vi "JAC_8216_Setting_Function_New.vi"(0 "JAC 8216_Control":T5, 1 "Initial":T4={"Card ID"=0, "IP_Address[4]"=[192, 168, 0, 100], "Hot post"=15122, "Remote port"=6936, "Time Out(ms)"=1000} {"Card ID" items=["0", "1", "2", "3", "4", "5", "6", "7", "8", "9", "10", "11", "12", "13", "14", "15", "16", "17", "18", "19", "20", "21", "22", "23", "24", "25", "26", "27", "28", "29", "30", "31", "32", "33", "34", "35", "36", "37", "38", "39", "40", "41", "42", "43", "44", "45", "46", "47", "48", "49", "50", "51", "52", "53", "54", "55", "56", "57", "58", "59", "60", "61", "62", "63", "64", "65", "66", "67", "68", "69", "70", "71", "72", "73", "74", "75", "76", "77", "78", "79", "80", "81", "82", "83", "84", "85", "86", "87", "88", "89", "90", "91", "92", "93", "94", "95", "96", "97", "98", "99", "100"]}, 2 "8216 IO In":T3, 3 "IO Polarity In":T1, 4 "IO Config In":T2 {"IO 17" items=["Output", "Input"]; "IO 16" items=["Output", "Input"]; "IO 15" items=["Output", "Input"]; "IO 14" items=["Output", "Input"]; "IO 13" items=["Output", "Input"]; "IO 12" items=["Output", "Input"]; "IO 11" items=["Output", "Input"]; "IO 10" items=["Output", "Input"]; "IO 07" items=["Output", "Input"]; "IO 06" items=["Output", "Input"]; "IO 05" items=["Output", "Input"]; "IO 04" items=["Output", "Input"]; "IO 03" items=["Output", "Input"]; "IO 02" items=["Output", "Input"]; "IO 01" items=["Output", "Input"]; "IO 00" items=["Output", "Input"]}, 5 "Error in":errorcluster) -> (15 "Port Status Out":bool[](array[boolean]), 16 "Input Out":u8, 17 "IO Polarity Out":T1, 18 "IO Config Out":T2 {"IO 17" items=["Output", "Input"]; "IO 16" items=["Output", "Input"]; "IO 15" items=["Output", "Input"]; "IO 14" items=["Output", "Input"]; "IO 13" items=["Output", "Input"]; "IO 12" items=["Output", "Input"]; "IO 11" items=["Output", "Input"]; "IO 10" items=["Output", "Input"]; "IO 07" items=["Output", "Input"]; "IO 06" items=["Output", "Input"]; "IO 05" items=["Output", "Input"]; "IO 04" items=["Output", "Input"]; "IO 03" items=["Output", "Input"]; "IO 02" items=["Output", "Input"]; "IO 01" items=["Output", "Input"]; "IO 00" items=["Output", "Input"]}, 19 "Error Out":errorcluster)   [LabVIEW 2015]
uses:
  JAC_8216_Control.ctl
  EMD8216_64/EMD8216_64.lvlib
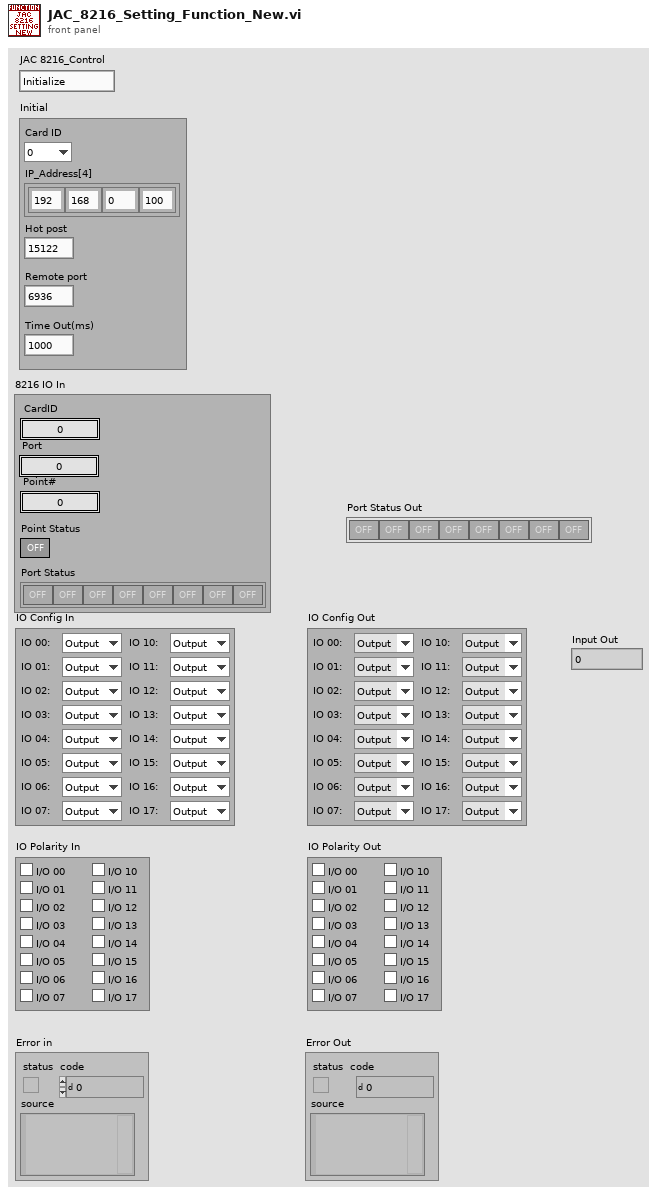
[diagram p1: front panel]
types:
  T1 = cluster{"IO 00":bool, "IO 01":bool, "IO 02":bool, "IO 03":bool, "IO 04":bool, "IO 05":bool, "IO 06":bool, "IO 07":bool, "IO 10":bool, "IO 11":bool, "IO 12":bool, "IO 13":bool, "IO 14":bool, "IO 15":bool, "IO 16":bool, "IO 17":bool}
  T2 = cluster{"IO 00":u8, "IO 01":u8, "IO 02":u8, "IO 03":u8, "IO 04":u8, "IO 05":u8, "IO 06":u8, "IO 07":u8, "IO 10":u8, "IO 11":u8, "IO 12":u8, "IO 13":u8, "IO 14":u8, "IO 15":u8, "IO 16":u8, "IO 17":u8}
  T3 = cluster{"CardID":u32, "Port":u8, "Point#":u8, "Point Status":bool, "Port Status":bool[]}
  T4 = cluster{"Card ID":u32, "IP_Address[4]":u8[], "Hot post":u16, "Remote port":u16, "Time Out(ms)":u16}
  T5 = typedef "JAC_8216_Control.ctl" = enum16{"Initialize", "Log Password", "Read IO Polarity ", "Set IO Polarity", "Read IO Config", "Set IO Config", "Read Input", "Set Output", "Read Port", "Close", "Idle"}
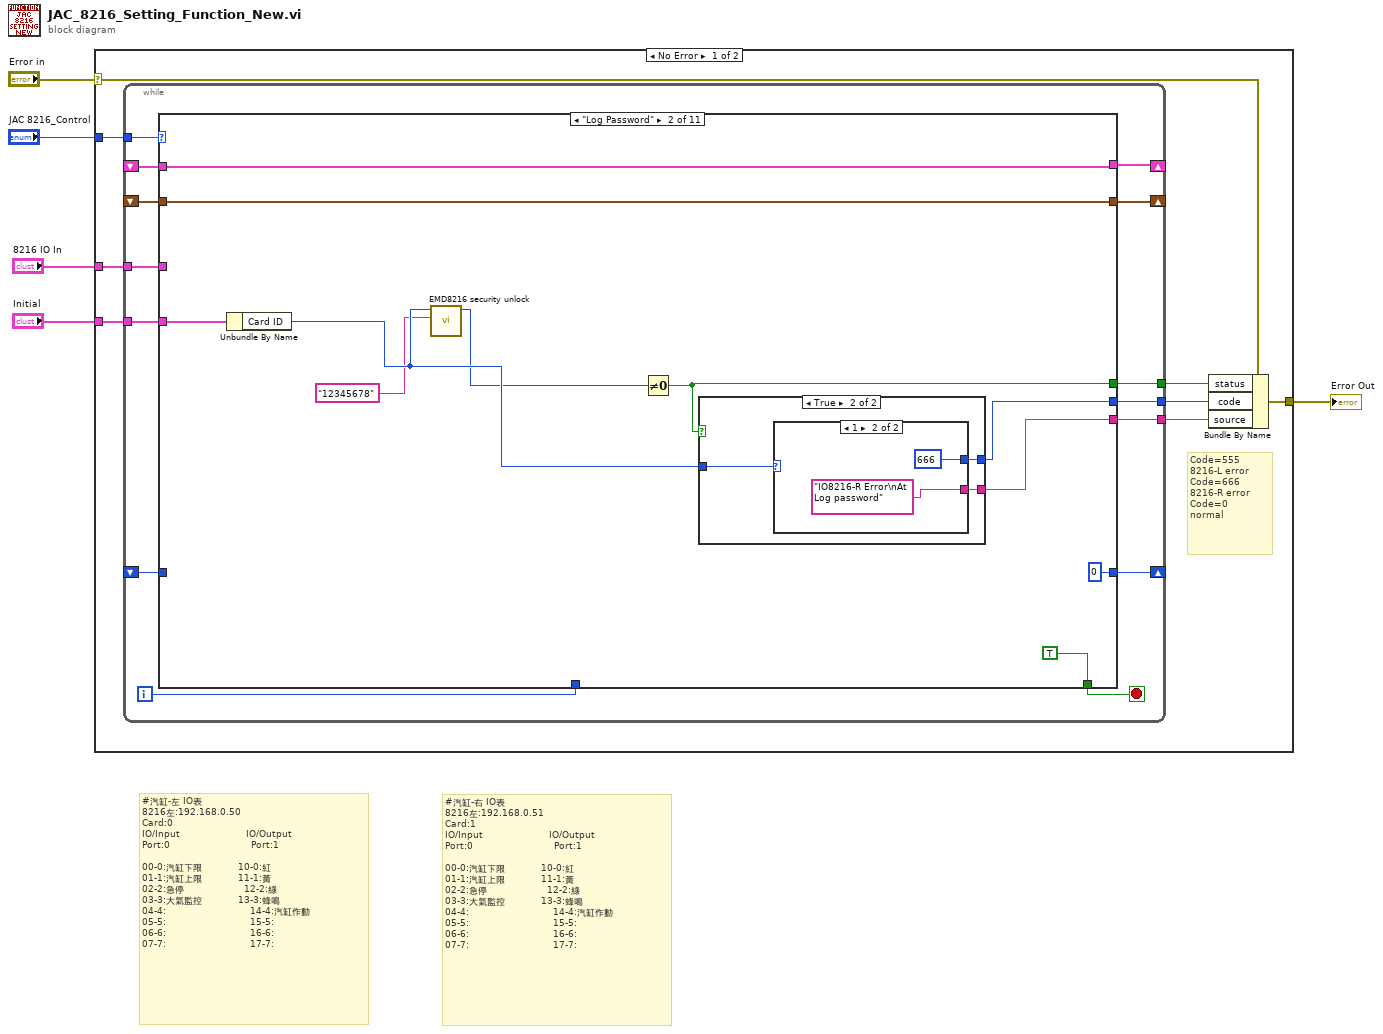
[diagram p0: block diagram]
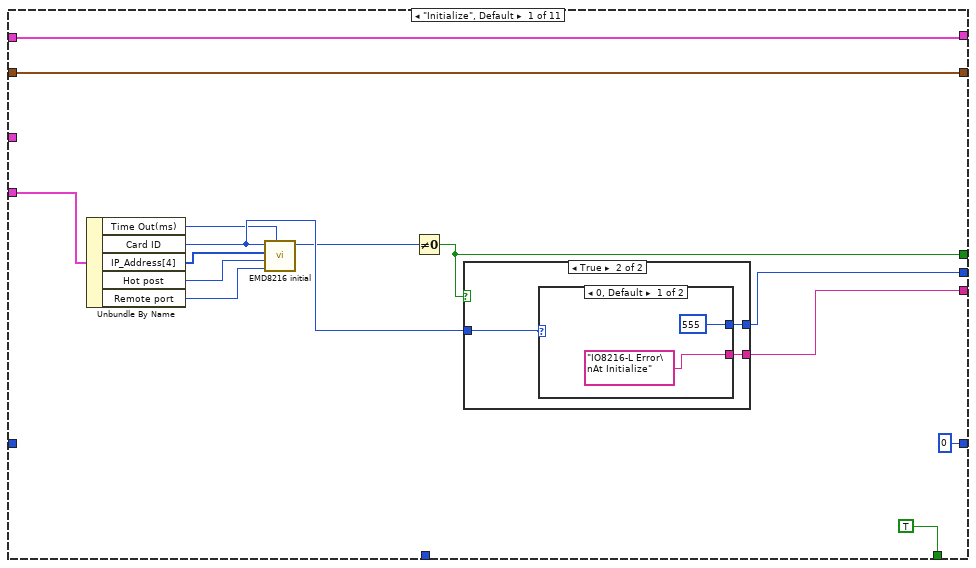
[diagram p2: hidden frame]
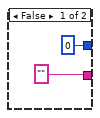
[diagram p3: hidden frame]
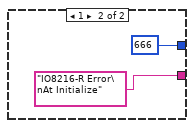
[diagram p4: hidden frame]
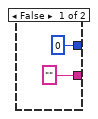
[diagram p5: hidden frame]
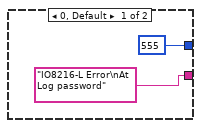
[diagram p6: hidden frame]
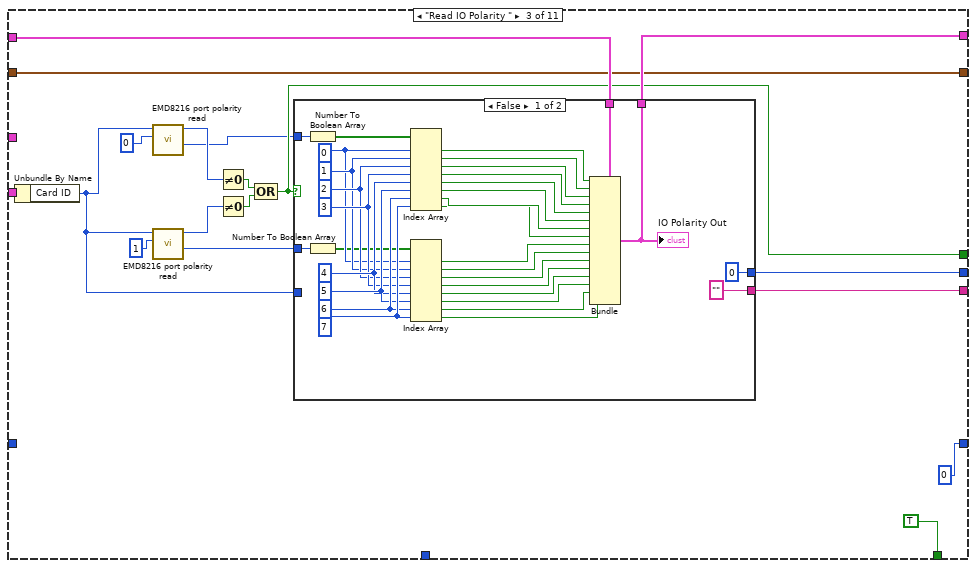
[diagram p7: hidden frame]
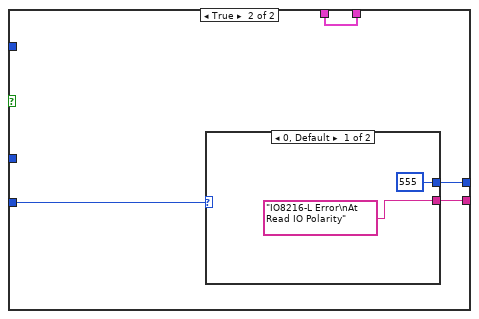
[diagram p8: hidden frame]
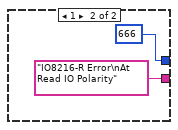
[diagram p9: hidden frame]
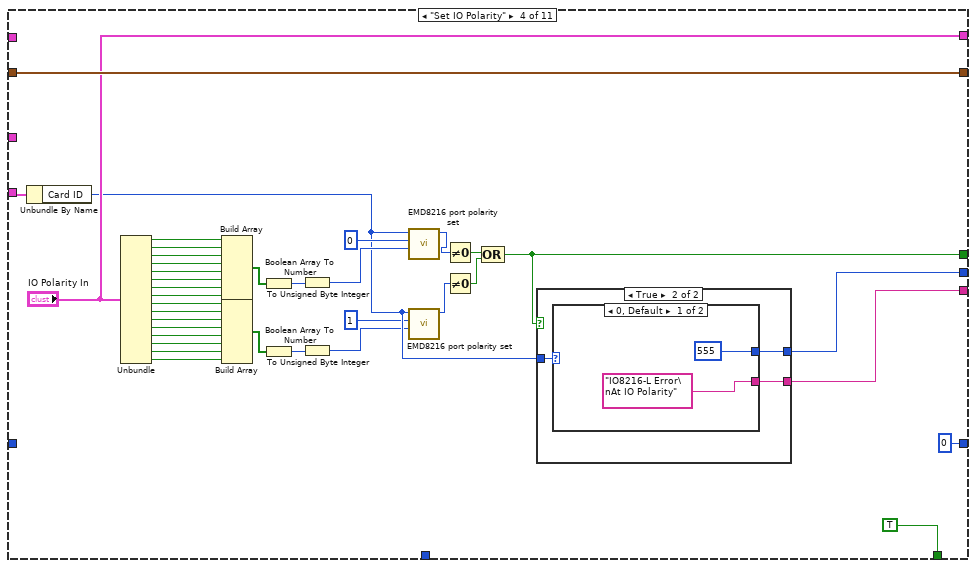
[diagram p10: hidden frame]
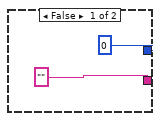
[diagram p11: hidden frame]
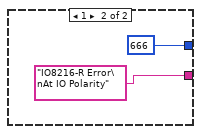
[diagram p12: hidden frame]
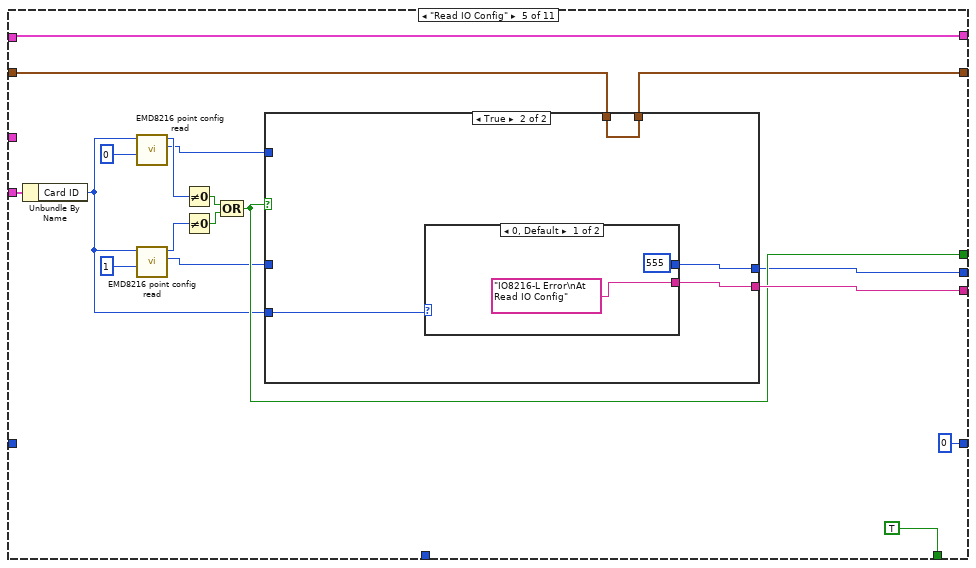
[diagram p13: hidden frame]
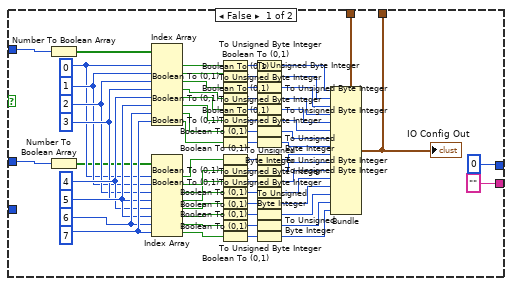
[diagram p14: hidden frame]
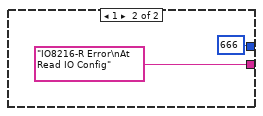
[diagram p15: hidden frame]
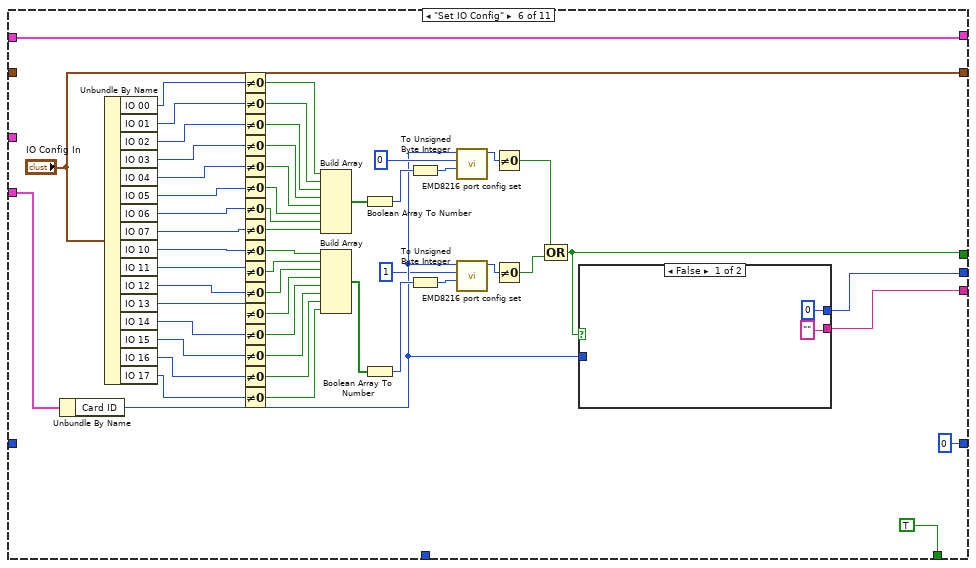
[diagram p16: hidden frame]
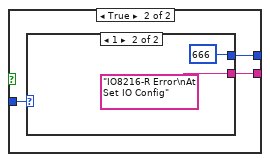
[diagram p17: hidden frame]
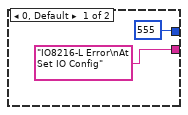
[diagram p18: hidden frame]
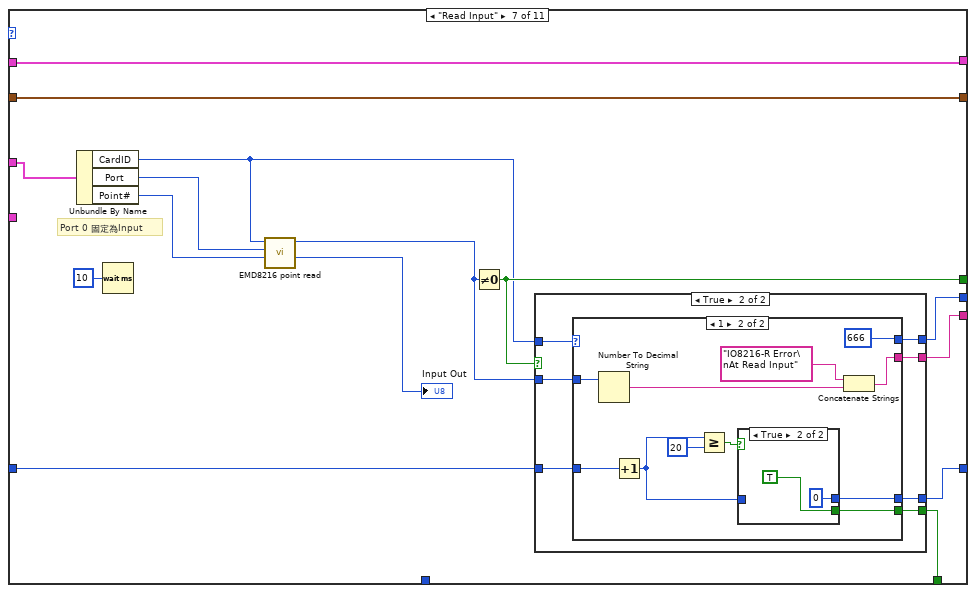
[diagram p19: hidden frame]
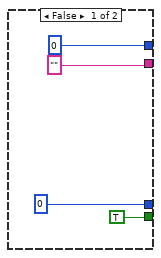
[diagram p20: hidden frame]
diagram:
  # "#汽缸-右 IO表\n8216左:192.168.0.51\nCard:1\nIO/Input                      IO/Output\nPort:0                           Port:1         \n         \n00-0:汽缸下限            10-0:紅   \n01-1:汽缸上限            11-1:黃\n02-2:急停                    12-2:綠\n03-3:大氣監控            13-3:蜂鳴\n04-4:                            14-4:汽缸作動\n05-5:                            15-5:\n06-6:                            16-6:\n07-7:                            17-7:"
  # "#汽缸-左 IO表\n8216左:192.168.0.50\nCard:0\nIO/Input                      IO/Output\nPort:0                           Port:1         \n         \n00-0:汽缸下限            10-0:紅   \n01-1:汽缸上限            11-1:黃\n02-2:急停                    12-2:綠\n03-3:大氣監控            13-3:蜂鳴\n04-4:                            14-4:汽缸作動\n05-5:                            15-5:\n06-6:                            16-6:\n07-7:                            17-7:"
  n1 = case shown="No Error" "Error in" {
    selector: "Error in" -> [w12 w490]
    tunnel: "JAC 8216_Control" -> [w13 _]
    tunnel: [w11 w490] -> w3
    tunnel: "Initial" -> [w10 _]
    tunnel: "8216 IO In" -> [w7 _]
    frame No Error {
      # "Code=555\n8216-L error\nCode=666\n8216-R error\nCode=0\nnormal"
      n2 = while {
        tunnel: w13 -> [w27]
        tunnel: w10 -> [w26]
        tunnel: [w25] -> w9
        tunnel: [w24] -> w8
        shift-right: [w23] -> _
        shift-left: _ -> [w22]
        shift-right: [w21] -> _
        shift-left: _ -> [w20]
        tunnel: w7 -> [w19]
        tunnel: [w18] -> w6
        shift-right: [w15] -> _
        shift-left: _ -> [w14]
        i -> [w17]
        stop <- w16 stop-if-true
        n3 = case shown="\"Log Password\"" w27 {
          tunnel: w26 -> [w41 w61 w83 w143 w192 w296 _ _ _ w473 _]
          tunnel: [w39 w58 w81 w140 w186 w276 w337 w394 w444 w470 FALSE] -> w25
          tunnel: [w40 w56 w82 w138 w187 w274 w336 w393 w445 w469 ""] -> w24
          tunnel: [w37 w59 w84 w165 w190 "IO Config In" w340 w399 w446 w471 w488] -> w23
          tunnel: w22 -> [w37 w59 w84 w165 w191 _ w340 w399 w446 w471 w488]
          tunnel: [w38 w60 w86 "IO Polarity In" w185 w278 w341 w400 w447 w472 w489] -> w21
          tunnel: w20 -> [w38 w60 w85 _ w185 w278 w341 w400 w447 w472 w489]
          tunnel: w19 -> [_ _ _ _ _ _ w339 w396 w442 _ _]
          tunnel: [w36 w57 w80 w139 w184 w275 w335 w392 w443 w468 0 ("code")] -> w18
          tunnel: w17 -> [_ _ _ _ _ _ _ w390 _ _ _]
          tunnel: [TRUE TRUE TRUE TRUE TRUE TRUE w333 w388 TRUE TRUE TRUE] -> w16
          tunnel: [0 0 0 0 0 0 w332 w391 0 0 0] -> w15
          tunnel: w14 -> [_ _ _ _ _ _ w334 w389 _ _ _]
          frame "Initialize", Default {
            n4 = Unbundle By Name(w41) -> ("Time Out(ms)"=w29:u16, "Card ID"=w33:u32, "IP_Address[4]"=w32:u8[], "Hot post"=w31:u16, "Remote port"=w30:u16)
            n5 = call "EMD8216 initial.vi"("TimeOut_ms"=w29, "Remote_port"=w30, "Host_Port"=w31, "IP_Address"=w32, "CardID"=w33) -> ("error_code"=w28:u32)  [unwired: 5 in, 1 out]
            n6 = Not Equal To 0?(x=w28) -> (x != 0?=w39:bool)
            n7 = case shown="True" w39 {
              tunnel: ["" w46] -> w40
              tunnel: w33 -> [_ w45]
              tunnel: [0 ("code") w44] -> w36
              frame False {
              }
              frame True {
                n8 = case shown="0, Default" w45 {
                  tunnel: ["IO8216-L Error\nAt Initialize" "IO8216-R Error\nAt Initialize"] -> w46
                  tunnel: [555 ("code") 666 ("code")] -> w44
                  frame 0, Default {
                  }
                  frame 1 {
                  }
                }
              }
            }
          }
          frame "Log Password" {
            n9 = Unbundle By Name(w61) -> ("Card ID"=w53:u32)
            n10 = call "EMD8216 security unlock.vi"("password"="12345678", "CardID"=w53) -> ("error_code"=w51:u32)  [unwired: 9 in]
            n11 = Not Equal To 0?(x=w51) -> (x != 0?=w58:bool)
            n12 = case shown="True" w58 {
              tunnel: ["" w66] -> w56
              tunnel: [0 ("code") w65] -> w57
              tunnel: w53 -> [_ w64]
              frame False {
              }
              frame True {
                n13 = case shown="1" w64 {
                  tunnel: ["IO8216-L Error\nAt Log password" "IO8216-R Error\nAt Log password"] -> w66
                  tunnel: [555 ("code") 666 ("code")] -> w65
                  frame 0, Default {
                  }
                  frame 1 {
                  }
                }
              }
            }
          }
          frame "Read IO Polarity " {
            n14 = Unbundle By Name(w83) -> ("Card ID"=w75:u32)
            n15 = call "EMD8216 port polarity read.vi"("port"=u8 0, "CardID"=w75) -> ("data"=w71:u8, "error_code"=w72:u32)  [unwired: 8 in]
            n16 = call "EMD8216 port polarity read.vi"("port"=u8 1, "CardID"=w75) -> ("data"=w74:u8, "error_code"=w73:u32)  [unwired: 8 in]
            n17 = Not Equal To 0?(x=w72) -> (x != 0?=w87:bool)
            n18 = Not Equal To 0?(x=w73) -> (x != 0?=w88:bool)
            n19 = Compound Arithmetic op=OR(w87, w88) -> (w81:bool)
            n20 = case shown="False" w81 {
              tunnel: [w107 w123] -> w86
              tunnel: w74 -> [w110 _]
              tunnel: w71 -> [w109 _]
              tunnel: ["" w124] -> w82
              tunnel: w85 -> [w90 w123]
              tunnel: w75 -> [_ w122]
              tunnel: [0 ("code") w121] -> w80
              frame False {
                w120 = 7
                w119 = 6
                w118 = 5
                w117 = 4
                w116 = 3
                w115 = 2
                w114 = 1
                w113 = 0
                n21 = Number To Boolean Array(number=w109) -> (Boolean array=w111:bool[])
                n22 = Number To Boolean Array(number=w110) -> (Boolean array=w112:bool[])
                n23 = Index Array(array=w111, index #1=w113, index #2=w114, index #3=w115, index #4=w116, index #5=w117, index #6=w118, index #7=w119, index #8=w120) -> (element #1=w106:bool, element #2=w105:bool, element #3=w104:bool, element #4=w103:bool, element #5=w102:bool, element #6=w101:bool, element #7=w100:bool, element #8=w99:bool)
                n24 = Index Array(array=w112, index #1=w113, index #2=w114, index #3=w115, index #4=w116, index #5=w117, index #6=w118, index #7=w119, index #8=w120) -> (element #1=w98:bool, element #2=w97:bool, element #3=w96:bool, element #4=w95:bool, element #5=w94:bool, element #6=w93:bool, element #7=w92:bool, element #8=w91:bool)
                n25 = Bundle(cluster=w90, "IO 00"=w106, "IO 01"=w105, "IO 02"=w104, "IO 03"=w103, "IO 04"=w102, "IO 05"=w101, "IO 06"=w100, "IO 07"=w99, "IO 10"=w98, "IO 11"=w97, "IO 12"=w96, "IO 13"=w95, "IO 14"=w94, "IO 15"=w93, "IO 16"=w92, "IO 17"=w91) -> (w107:T1)
                "IO Polarity Out" <- w107
              }
              frame True {
                n26 = case shown="0, Default" w122 {
                  tunnel: ["IO8216-L Error\nAt Read IO Polarity" "IO8216-R Error\nAt Read IO Polarity"] -> w124
                  tunnel: [555 ("code") 666 ("code")] -> w121
                  frame 0, Default {
                  }
                  frame 1 {
                  }
                }
              }
            }
          }
          frame "Set IO Polarity" {
            n27 = Unbundle By Name(w143) -> ("Card ID"=w132:u32)
            n28 = Unbundle("IO Polarity In") -> ("IO 00"=w159:bool, "IO 01"=w158:bool, "IO 02"=w157:bool, "IO 03"=w156:bool, "IO 04"=w155:bool, "IO 05"=w154:bool, "IO 06"=w153:bool, "IO 07"=w152:bool, "IO 10"=w151:bool, "IO 11"=w150:bool, "IO 12"=w149:bool, "IO 13"=w148:bool, "IO 14"=w147:bool, "IO 15"=w146:bool, "IO 16"=w145:bool, "IO 17"=w144:bool)
            n29 = Build Array(w159, w158, w157, w156, w155, w154, w153, w152) -> (w163:bool[])
            n30 = Build Array(w151, w150, w149, w148, w147, w146, w145, w144) -> (w161:bool[])
            n31 = Boolean Array To Number(Boolean array=w163) -> (number=w162:u32)
            n32 = Boolean Array To Number(Boolean array=w161) -> (number=w160:u32)
            n33 = To Unsigned Byte Integer(number=w162) -> (unsigned 8bit integer=w134:u8)
            n34 = To Unsigned Byte Integer(number=w160) -> (unsigned 8bit integer=w130:u8)
            n35 = call "EMD8216 port polarity set.vi"("data"=w134, "port"=u8 0, "CardID"=w132) -> ("error_code"=w133:u32)  [unwired: 8 in]
            n36 = call "EMD8216 port polarity set.vi"("data"=w130, "port"=u8 1, "CardID"=w132) -> ("error_code"=w129:u32)  [unwired: 8 in]
            n37 = Not Equal To 0?(x=w133) -> (x != 0?=w141:bool)
            n38 = Not Equal To 0?(x=w129) -> (x != 0?=w142:bool)
            n39 = Compound Arithmetic op=OR(w141, w142) -> (w140:bool)
            n40 = case shown="True" w140 {
              tunnel: ["" w170] -> w138
              tunnel: [0 ("code") w169] -> w139
              tunnel: w132 -> [_ w168]
              frame False {
              }
              frame True {
                n41 = case shown="0, Default" w168 {
                  tunnel: ["IO8216-L Error\nAt IO Polarity" "IO8216-R Error\nAt IO Polarity"] -> w170
                  tunnel: [555 ("code") 666 ("code")] -> w169
                  frame 0, Default {
                  }
                  frame 1 {
                  }
                }
              }
            }
          }
          frame "Read IO Config" {
            n42 = Unbundle By Name(w192) -> ("Card ID"=w177:u32)
            n43 = call "EMD8216 point config read.vi"("point"=u8 0, "CardID"=w177) -> ("config"=w179:u8, "error_code"=w180:u32)  [unwired: 8 in]
            n44 = call "EMD8216 point config read.vi"("point"=u8 1, "CardID"=w177) -> ("config"=w175:u8, "error_code"=w176:u32)  [unwired: 8 in]
            n45 = Not Equal To 0?(x=w180) -> (x != 0?=w188:bool)
            n46 = Not Equal To 0?(x=w176) -> (x != 0?=w189:bool)
            n47 = Compound Arithmetic op=OR(w188, w189) -> (w186:bool)
            n48 = case shown="True" w186 {
              tunnel: w191 -> [w256 w260]
              tunnel: [w255 w260] -> w190
              tunnel: w175 -> [w212 _]
              tunnel: w179 -> [w211 _]
              tunnel: ["" w259] -> w187
              tunnel: w177 -> [_ w258]
              tunnel: [0 w257] -> w184
              frame False {
                w222 = 7
                w221 = 6
                w220 = 5
                w219 = 4
                w218 = 3
                w217 = 2
                w216 = 1
                w215 = 0
                n49 = Number To Boolean Array(number=w211) -> (Boolean array=w213:bool[])
                n50 = Number To Boolean Array(number=w212) -> (Boolean array=w214:bool[])
                n51 = Index Array(array=w213, index #1=w215, index #2=w216, index #3=w217, index #4=w218, index #5=w219, index #6=w220, index #7=w221, index #8=w222) -> (element #1=w254:bool, element #2=w252:bool, element #3=w251:bool, element #4=w250:bool, element #5=w249:bool, element #6=w248:bool, element #7=w247:bool, element #8=w246:bool)
                n52 = Index Array(array=w214, index #1=w215, index #2=w216, index #3=w217, index #4=w218, index #5=w219, index #6=w220, index #7=w221, index #8=w222) -> (element #1=w245:bool, element #2=w244:bool, element #3=w243:bool, element #4=w242:bool, element #5=w241:bool, element #6=w240:bool, element #7=w239:bool, element #8=w238:bool)
                n53 = Boolean To (0,1)(Boolean=w254) -> (0, 1=w253:i16)
                n54 = Boolean To (0,1)(Boolean=w252) -> (0, 1=w223:i16)
                n55 = Boolean To (0,1)(Boolean=w251) -> (0, 1=w225:i16)
                n56 = Boolean To (0,1)(Boolean=w250) -> (0, 1=w224:i16)
                n57 = Boolean To (0,1)(Boolean=w249) -> (0, 1=w229:i16)
                n58 = Boolean To (0,1)(Boolean=w248) -> (0, 1=w228:i16)
                n59 = Boolean To (0,1)(Boolean=w247) -> (0, 1=w226:i16)
                n60 = Boolean To (0,1)(Boolean=w246) -> (0, 1=w227:i16)
                n61 = Boolean To (0,1)(Boolean=w245) -> (0, 1=w237:i16)
                n62 = Boolean To (0,1)(Boolean=w244) -> (0, 1=w236:i16)
                n63 = Boolean To (0,1)(Boolean=w243) -> (0, 1=w234:i16)
                n64 = Boolean To (0,1)(Boolean=w242) -> (0, 1=w235:i16)
                n65 = Boolean To (0,1)(Boolean=w241) -> (0, 1=w230:i16)
                n66 = Boolean To (0,1)(Boolean=w240) -> (0, 1=w231:i16)
                n67 = Boolean To (0,1)(Boolean=w239) -> (0, 1=w233:i16)
                n68 = Boolean To (0,1)(Boolean=w238) -> (0, 1=w232:i16)
                n69 = To Unsigned Byte Integer(number=w253) -> (unsigned 8bit integer=w210:u8)
                n70 = To Unsigned Byte Integer(number=w223) -> (unsigned 8bit integer=w209:u8)
                n71 = To Unsigned Byte Integer(number=w225) -> (unsigned 8bit integer=w208:u8)
                n72 = To Unsigned Byte Integer(number=w224) -> (unsigned 8bit integer=w207:u8)
                n73 = To Unsigned Byte Integer(number=w229) -> (unsigned 8bit integer=w206:u8)
                n74 = To Unsigned Byte Integer(number=w228) -> (unsigned 8bit integer=w205:u8)
                n75 = To Unsigned Byte Integer(number=w226) -> (unsigned 8bit integer=w204:u8)
                n76 = To Unsigned Byte Integer(number=w227) -> (unsigned 8bit integer=w203:u8)
                n77 = To Unsigned Byte Integer(number=w237) -> (unsigned 8bit integer=w202:u8)
                n78 = To Unsigned Byte Integer(number=w236) -> (unsigned 8bit integer=w201:u8)
                n79 = To Unsigned Byte Integer(number=w234) -> (unsigned 8bit integer=w200:u8)
                n80 = To Unsigned Byte Integer(number=w235) -> (unsigned 8bit integer=w199:u8)
                n81 = To Unsigned Byte Integer(number=w230) -> (unsigned 8bit integer=w198:u8)
                n82 = To Unsigned Byte Integer(number=w231) -> (unsigned 8bit integer=w197:u8)
                n83 = To Unsigned Byte Integer(number=w233) -> (unsigned 8bit integer=w196:u8)
                n84 = To Unsigned Byte Integer(number=w232) -> (unsigned 8bit integer=w195:u8)
                n85 = Bundle(cluster=w256, "IO 00"=w210, "IO 01"=w209, "IO 02"=w208, "IO 03"=w207, "IO 04"=w206, "IO 05"=w205, "IO 06"=w204, "IO 07"=w203, "IO 10"=w202, "IO 11"=w201, "IO 12"=w200, "IO 13"=w199, "IO 14"=w198, "IO 15"=w197, "IO 16"=w196, "IO 17"=w195) -> (w255:T2)
                "IO Config Out" <- w255
              }
              frame True {
                n86 = case shown="0, Default" w258 {
                  tunnel: ["IO8216-L Error\nAt Read IO Config" "IO8216-R Error\nAt Read IO Config"] -> w259
                  tunnel: [555 666] -> w257
                  frame 0, Default {
                  }
                  frame 1 {
                  }
                }
              }
            }
          }
          frame "Set IO Config" {
            n87 = Unbundle By Name(w296) -> ("Card ID"=w268:u32)
            n88 = Unbundle By Name("IO Config In") -> ("IO 00"=w297:u8, "IO 01"=w295:u8, "IO 02"=w294:u8, "IO 03"=w293:u8, "IO 04"=w292:u8, "IO 05"=w291:u8, "IO 06"=w290:u8, "IO 07"=w289:u8, "IO 10"=w281:u8, "IO 11"=w282:u8, "IO 12"=w283:u8, "IO 13"=w284:u8, "IO 14"=w285:u8, "IO 15"=w286:u8, "IO 16"=w287:u8, "IO 17"=w288:u8)
            n89 = Not Equal To 0?(x=w297) -> (x != 0?=w316:bool)
            n90 = Not Equal To 0?(x=w295) -> (x != 0?=w315:bool)
            n91 = Not Equal To 0?(x=w294) -> (x != 0?=w314:bool)
            n92 = Not Equal To 0?(x=w293) -> (x != 0?=w313:bool)
            n93 = Not Equal To 0?(x=w292) -> (x != 0?=w305:bool)
            n94 = Not Equal To 0?(x=w291) -> (x != 0?=w304:bool)
            n95 = Not Equal To 0?(x=w290) -> (x != 0?=w303:bool)
            n96 = Not Equal To 0?(x=w289) -> (x != 0?=w302:bool)
            n97 = Not Equal To 0?(x=w281) -> (x != 0?=w309:bool)
            n98 = Not Equal To 0?(x=w282) -> (x != 0?=w308:bool)
            n99 = Not Equal To 0?(x=w283) -> (x != 0?=w307:bool)
            n100 = Not Equal To 0?(x=w284) -> (x != 0?=w317:bool)
            n101 = Not Equal To 0?(x=w285) -> (x != 0?=w306:bool)
            n102 = Not Equal To 0?(x=w286) -> (x != 0?=w301:bool)
            n103 = Not Equal To 0?(x=w287) -> (x != 0?=w300:bool)
            n104 = Not Equal To 0?(x=w288) -> (x != 0?=w299:bool)
            n105 = Build Array(w316, w315, w314, w313, w305, w304, w303, w302) -> (w312:bool[])
            n106 = Build Array(w309, w308, w307, w317, w306, w301, w300, w299) -> (w298:bool[])
            n107 = Boolean Array To Number(Boolean array=w312) -> (number=w311:u32)
            n108 = Boolean Array To Number(Boolean array=w298) -> (number=w310:u32)
            n109 = To Unsigned Byte Integer(number=w311) -> (unsigned 8bit integer=w270:u8)
            n110 = To Unsigned Byte Integer(number=w310) -> (unsigned 8bit integer=w266:u8)
            n111 = call "EMD8216 port config set.vi"("config"=w270, "port"=u8 0, "CardID"=w268) -> ("error_code"=w269:u32)  [unwired: 8 in]
            n112 = call "EMD8216 port config set.vi"("config"=w266, "port"=u8 1, "CardID"=w268) -> ("error_code"=w265:u32)  [unwired: 8 in]
            n113 = Not Equal To 0?(x=w269) -> (x != 0?=w280:bool)
            n114 = Not Equal To 0?(x=w265) -> (x != 0?=w279:bool)
            n115 = Compound Arithmetic op=OR(w280, w279) -> (w276:bool)
            n116 = case shown="False" w276 {
              tunnel: w268 -> [_ w322]
              tunnel: [0 w321] -> w275
              tunnel: ["" w320] -> w274
              frame False {
              }
              frame True {
                n117 = case shown="1" w322 {
                  tunnel: ["IO8216-L Error\nAt Set IO Config" "IO8216-R Error\nAt Set IO Config"] -> w320
                  tunnel: [555 666] -> w321
                  frame 0, Default {
                  }
                  frame 1 {
                  }
                }
              }
            }
          }
          frame "Read Input" {
            # "Port 0 固定為Input"
            n118 = Unbundle By Name(w339) -> ("CardID"=w331:u32, "Port"=w330:u8, "Point#"=w329:u8)
            n119 = Wait (ms)(milliseconds to wait=u32 10) -> ()  [unwired: 1 out]
            n120 = call "EMD8216 point read.vi"("point"=w329, "port"=w330, "CardID"=w331) -> ("state"=→"Input Out":u8, "error_code"=w328:u32)  [unwired: 7 in]
            n121 = Not Equal To 0?(x=w328) -> (x != 0?=w337:bool)
            n122 = case shown="True" w337 {
              tunnel: [0 w352] -> w335
              tunnel: ["" w351] -> w336
              tunnel: w331 -> [_ w350]
              tunnel: w328 -> [_ w349]
              tunnel: w334 -> [_ w348]
              tunnel: [TRUE w347] -> w333
              tunnel: [0 w346] -> w332
              frame False {
              }
              frame True {
                n123 = case shown="1" w350 {
                  tunnel: [w359 w376] -> w351
                  tunnel: [555 666] -> w352
                  tunnel: w349 -> [w360 w377]
                  tunnel: w348 -> [w355 w370]
                  tunnel: [w353 w369] -> w347
                  tunnel: [w354 w368] -> w346
                  frame 0, Default {
                    n124 = Increment(x=w355) -> (x+1=w357:i32)
                    n125 = Number To Decimal String(number=w360) -> (decimal integer string=w361:string)  [unwired: 1 in]
                    n126 = Greater Or Equal?(x=w357, y=20) -> (x >= y?=w358:bool)
                    n127 = case shown="True" w358 {
                      tunnel: [w365 w367] -> w354
                      tunnel: w357 -> [w365 w367]
                      tunnel: [FALSE TRUE] -> w353
                      frame False {
                      }
                      frame True {
                      }
                    }
                    n128 = Concatenate Strings("IO8216-L Error\nAt Read Input", w361) -> (w359:string)
                  }
                  frame 1 {
                    n129 = Number To Decimal String(number=w377) -> (decimal integer string=w374:string)  [unwired: 1 in]
                    n130 = Increment(x=w370) -> (x+1=w372:i32)
                    n131 = Greater Or Equal?(x=w372, y=20) -> (x >= y?=w373:bool)
                    n132 = case shown="True" w373 {
                      tunnel: [w380 0] -> w368
                      tunnel: w372 -> [w380 _]
                      tunnel: [FALSE TRUE] -> w369
                      frame False {
                      }
                      frame True {
                      }
                    }
                    n133 = Concatenate Strings("IO8216-R Error\nAt Read Input", w374) -> (w376:string)
                  }
                }
              }
            }
          }
          frame "Set Output" {
            # "Port 1 固定為OutPut"
            n134 = Wait (ms)(milliseconds to wait=u32 10) -> ()  [unwired: 1 out]
            n135 = Unbundle By Name(w396) -> ("CardID"=w387:u32, "Port"=w386:u8, "Point#"=w385:u8, "Point Status"=w397:bool)
            n136 = Boolean To (0,1)(Boolean=w397) -> (0, 1=w398:i16)
            n137 = To Unsigned Byte Integer(number=w398) -> (unsigned 8bit integer=w384:u8)
            n138 = call "EMD8216 point set.vi"("state"=w384, "point"=w385, "port"=w386, "CardID"=w387) -> ("error_code"=w383:u32)  [unwired: 7 in]
            n139 = Not Equal To 0?(x=w383) -> (x != 0?=w394:bool)
            n140 = case shown="True" w394 {
              tunnel: [0 w410] -> w392
              tunnel: ["" w409] -> w393
              tunnel: w387 -> [_ w408]
              tunnel: [0 w406] -> w391
              tunnel: w390 -> [_ _]
              tunnel: w389 -> [_ w407]
              tunnel: [TRUE w405] -> w388
              frame False {
              }
              frame True {
                n141 = case shown="0, Default" w408 {
                  tunnel: ["IO8216-L Error\nAt Set Output" "IO8216-R Error\nAt Set Output"] -> w409
                  tunnel: [555 666] -> w410
                  tunnel: w407 -> [w413 w428]
                  tunnel: [w412 w427] -> w406
                  tunnel: [w411 w423] -> w405
                  frame 0, Default {
                    n142 = Increment(x=w413) -> (x+1=w415:i32)
                    n143 = Greater Or Equal?(x=w415, y=20) -> (x >= y?=w416:bool)
                    n144 = case shown="False" w416 {
                      tunnel: [w420 w422] -> w412
                      tunnel: w415 -> [w420 w422]
                      tunnel: [FALSE TRUE] -> w411
                      frame False {
                      }
                      frame True {
                      }
                    }
                  }
                  frame 1 {
                    n145 = Increment(x=w428) -> (x+1=w425:i32)
                    n146 = Greater Or Equal?(x=w425, y=20) -> (x >= y?=w426:bool)
                    n147 = case shown="False" w426 {
                      tunnel: [w432 w434] -> w427
                      tunnel: w425 -> [w432 w434]
                      tunnel: [FALSE TRUE] -> w423
                      frame False {
                      }
                      frame True {
                      }
                    }
                  }
                }
              }
            }
          }
          frame "Read Port" {
            n148 = Unbundle By Name(w442) -> ("CardID"=w438:u32, "Port"=w437:u8)
            n149 = call "EMD8216 port read.vi"("port"=w437, "CardID"=w438) -> ("data"=w435:u8, "error_code"=w436:u32)  [unwired: 8 in]
            n150 = Not Equal To 0?(x=w436) -> (x != 0?=w444:bool)
            n151 = case shown="True" w444 {
              tunnel: [0 w453] -> w443
              tunnel: ["" w452] -> w445
              tunnel: w438 -> [_ w451]
              tunnel: w436 -> [_ w450]
              frame False {
              }
              frame True {
                n152 = case shown="0, Default" w451 {
                  tunnel: [w454 w459] -> w452
                  tunnel: [555 666] -> w453
                  tunnel: w450 -> [w457 w461]
                  frame 0, Default {
                    n153 = Number To Decimal String(number=w457) -> (decimal integer string=w456:string)  [unwired: 1 in]
                    n154 = Concatenate Strings(w456, "IO8216-L Error\nAt Read Port") -> (w454:string)
                  }
                  frame 1 {
                    n155 = Number To Decimal String(number=w461) -> (decimal integer string=w462:string)  [unwired: 1 in]
                    n156 = Concatenate Strings(w462, "IO8216-R Error\nAt Read Port") -> (w459:string)
                  }
                }
              }
            }
            n157 = Number To Boolean Array(number=w435) -> (Boolean array=→"Port Status Out":bool[])
          }
          frame "Close" {
            n158 = Unbundle By Name(w473) -> ("Card ID"=w465:u32)
            n159 = call "EMD8216 close.vi"("CardID"=w465) -> ("error_code"=w464:u32)  [unwired: 10 in]
            n160 = Not Equal To 0?(x=w464) -> (x != 0?=w470:bool)
            n161 = case shown="True" w470 {
              tunnel: ["" w478] -> w469
              tunnel: w465 -> [_ w477]
              tunnel: [0 w476] -> w468
              frame False {
              }
              frame True {
                n162 = case shown="0, Default" w477 {
                  tunnel: ["IO8216-L Error\nAt Close" "IO8216-R Error\nAt Close"] -> w478
                  tunnel: [555 666] -> w476
                  frame 0, Default {
                  }
                  frame 1 {
                  }
                }
              }
            }
          }
          frame "Idle" {
          }
        }
      }
      n163 = Bundle By Name(cluster=w12, "status"=w9, "code"=w6, "source"=w8) -> (w11:errorcluster)
    }
    frame Error {
    }
  }
  "Error Out" <- w3
